vi "PRIME Detector Start Python Server.vi"(8 "error in (no error)":errorcluster, 11 "working directory":path=path "") -> (0 "error out":errorcluster, 2 "return code":i32, 3 "standard output":string)   [LabVIEW 2021, in "PRIME Detector.lvclass"]
uses:
  PRIME Detector.lvclass
  31452220-4626-403b-a302-208ddba39589.vi
panel:
  out "standard error":string
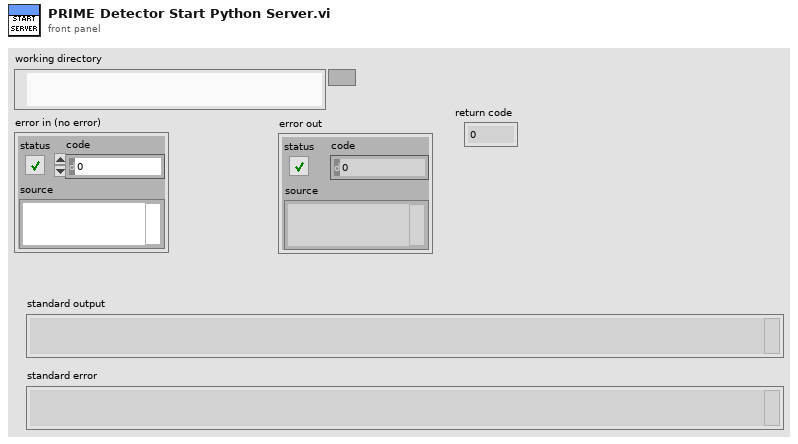
[diagram p1: front panel]
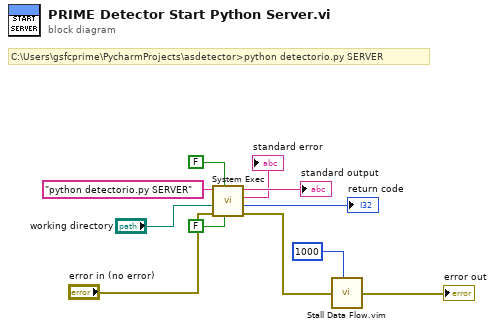
[diagram p0: block diagram]
diagram:
  # "C:\\Users\\gsfcprime\\PycharmProjects\\asdetector>python detectorio.py SERVER"
  n1 = call <vilib>:"System Exec.vi"("run minimized? (F)"=FALSE, "wait until completion? (T)"=FALSE, "error in (no error)"="error in (no error)", "working directory"="working directory", "command line"="python detectorio.py SERVER") -> ("error out"=w7:errorcluster, "return code"=→"return code":i32, "standard error"=→"standard error":string, "standard output"=→"standard output":string)  [unwired: 3 in]
  n2 = call "Stall Data Flow.vim"("value in"=w7, "milliseconds to wait"=u32 1000) -> ("value out"=→"error out":errorcluster)  [unwired: 1 out]
